vi "Reduce Path.vi"(11 "Path in":i32[][](array[numeric])) -> (3 "Reduced Path":i32[][](array[numeric]))   [LabVIEW 2012]
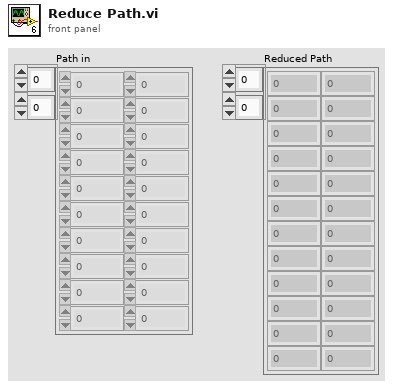
[diagram p1: front panel]
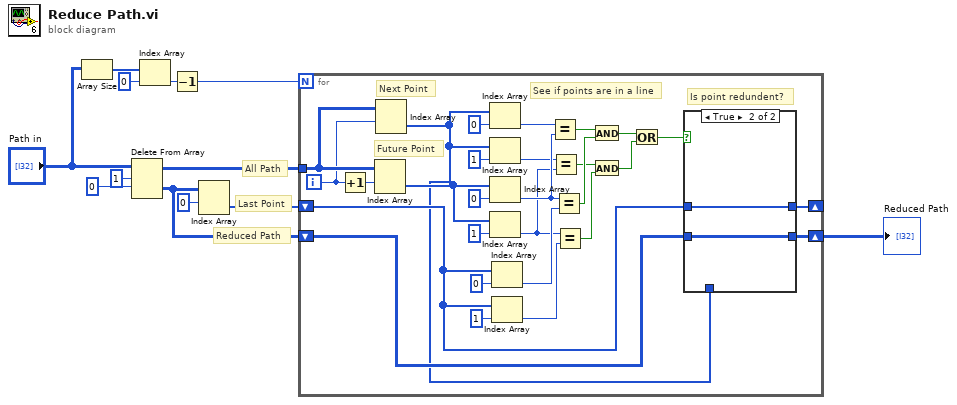
[diagram p0: block diagram]
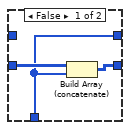
[diagram p2: hidden frame]
diagram:
  # "Reduced Path"
  # "Last Point"
  # "All Path"
  n1 = Array Size(array="Path in") -> (size(s)=w12:i32[])
  n2 = Delete From Array(array="Path in", length=1, index (row)=0) -> (deleted portion=w3:i32[][], array with subset deleted=w5:i32[][])  [unwired: 1 in]
  n3 = Index Array(array=w12, index=0) -> (element=w10:i32)
  n4 = Decrement(x=w10) -> (x-1=w9:i32)
  n5 = Index Array(array=w3, index (row)=0 ("index")) -> (element=w2:i32[])  [unwired: 1 in]
  n6 = for {
    N: w9 -> [_]
    shift-right: [w15] -> w8
    shift-left: w3 -> [w14]
    tunnel: w5 -> [w40]
    shift-right: [w17] -> _
    shift-left: w2 -> [w16]
    i -> [w39]
    # "Is point redundent?"
    # "See if points are in a line"
    # "Future Point"
    # "Next Point"
    n7 = Increment(x=w39) -> (x+1=w38:i32)
    n8 = Index Array(array=w40, index (row)=w38) -> (element=w35:i32[])  [unwired: 1 in]
    n9 = Index Array(array=w40, index (row)=w39) -> (element=w13:i32[])  [unwired: 1 in]
    n10 = Index Array(array=w13, index=0) -> (element=w29:i32)
    n11 = Index Array(array=w13, index=1) -> (element=w23:i32)
    n12 = Index Array(array=w35, index=0) -> (element=w28:i32)
    n13 = Index Array(array=w35, index=1) -> (element=w22:i32)
    n14 = Index Array(array=w16, index=0) -> (element=w30:i32)
    n15 = Index Array(array=w16, index=1) -> (element=w21:i32)
    n16 = Equal?(x=w29, y=w28) -> (x = y?=w27:bool)
    n17 = Equal?(x=w23, y=w22) -> (x = y?=w24:bool)
    n18 = Equal?(x=w28, y=w30) -> (x = y?=w26:bool)
    n19 = Equal?(x=w22, y=w21) -> (x = y?=w25:bool)
    n20 = And(x=w27, y=w26) -> (x .and. y?=w20:bool)
    n21 = And(x=w24, y=w25) -> (x .and. y?=w19:bool)
    n22 = Or(x=w20, y=w19) -> (x .or. y?=w18:bool)
    n23 = case shown="True" w18 {
      tunnel: [w41 w45] -> w17
      tunnel: w16 -> [_ w45]
      tunnel: [w42 w44] -> w15
      tunnel: w14 -> [w43 w44]
      tunnel: w13 -> [w41 _]
      frame False {
        n24 = Build Array (concatenate)(w43, w41) -> (w42:i32[][])
      }
      frame True {
      }
    }
  }
  "Reduced Path" <- w8
